vi "Polynomentwicklung Array IAG.vi"(9 "P(x) 2":dbl[](array[numeric]) caption="P(x)" min=0.0 max=127.0 format="%#.2f", 11 "A":dbl[](array[numeric])) -> (3 "P(A)":dbl[](array[numeric]))   [LabVIEW 2020, in "Linearisierung v2.lvlib"]
uses:
  Linearisierung v2.lvlib
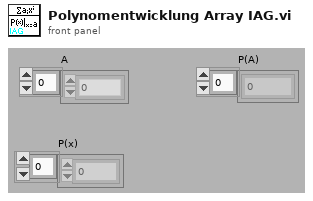
[diagram p1: front panel]
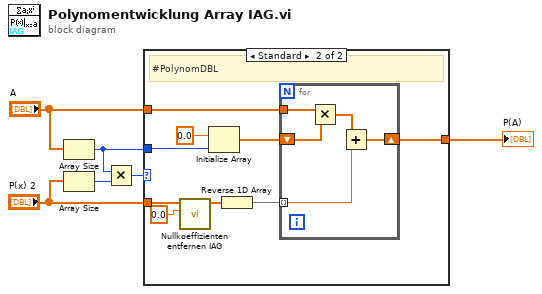
[diagram p0: block diagram]
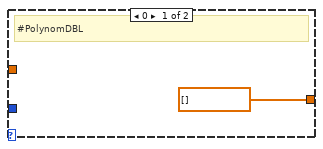
[diagram p2: hidden frame]
diagram:
  n1 = Array Size(array="A") -> (size(s)=w6:i32)
  n2 = Array Size(array="P(x) 2") -> (size(s)=w3:i32)
  n3 = Multiply(x=w6, y=w3) -> (x*y=w4:i32)
  n4 = case shown="Standard" w4 {
    tunnel: "P(x) 2" -> [_ w10]
    tunnel: "A" -> [_ w15]
    tunnel: [dbl[] [] w14] -> w1
    tunnel: w6 -> [_ w12]
    frame 0 {
      # "#PolynomDBL"
    }
    frame Default {
      # "#PolynomDBL"
      n5 = call "Nullkoeffizienten entfernen IAG.vi"("threshold"=0.0, "P(x) In"=w10) -> ("P(x) Out"=w8:dbl[])  [unwired: 8 in, 1 out]
      n6 = Initialize Array(0.0, w12) -> (w11:dbl[])
      n7 = Reverse 1D Array(array=w8) -> (reversed array=w16:dbl[])
      n8 = for {
        shift-right: [w17] -> w14
        shift-left: w11 -> [w20]
        tunnel: w15 -> [w21]
        tunnel: w16 -> [w19] mode=indexing
        n9 = Multiply(x=w21, y=w20) -> (x*y=w18:dbl[])
        n10 = Add(x=w18, y=w19) -> (x+y=w17:dbl[])
      }
    }
  }
  "P(A)" <- w1
